vi "Position Data.vi"() -> ()   [LabVIEW 2017]
panel:
  in  "Path Name":string
  out "Zero XY?":bool
  out "X position":dbl
  out "Y position":dbl
  out "IMU Heading":dbl
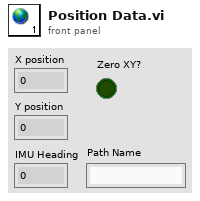
[diagram p1: front panel]
diagram:
